vi "moveStageREL_xy.vi"(4 "Radio Buttons":enum32{"Coarse (mm) ", "Fine (um) "}(radio)=enum."Fine (um) ", 5 "increment":dbl, 6 "initPos (mm)":dbl, 7 "stage lim (mm)":dbl, 8 "axisIdx":i32, 9 "System no.":i32=1 min=1 max=4 step=1, 10 "stageInit":i16) -> (2 "finPos":dbl)   [LabVIEW 2015]
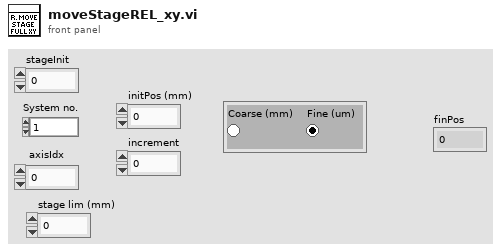
[diagram p1: front panel]
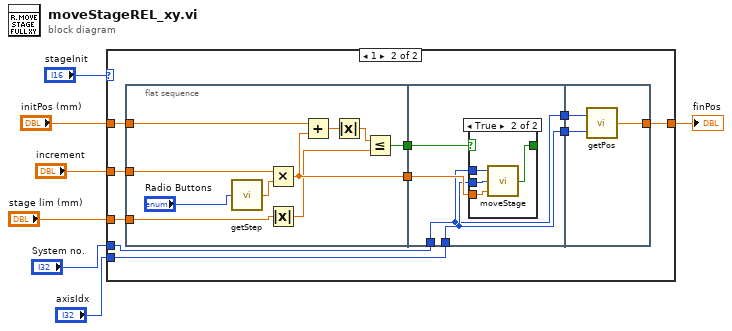
[diagram p0: block diagram]
diagram:
  n1 = case shown="1" "stageInit" {
    tunnel: [w8 w16] -> w7
    tunnel: "initPos (mm)" -> [w8 w13]
    tunnel: "System no." -> [_ w15]
    tunnel: "axisIdx" -> [_ w14]
    tunnel: "increment" -> [_ w12]
    tunnel: "stage lim (mm)" -> [_ w9]
    frame 0, Default {
    }
    frame 1 {
      n2 = flat-sequence {
        tunnel: [w27] -> w18
        tunnel: [w26] -> w17
        tunnel: w13 -> [w21]
        tunnel: w12 -> [w20]
        tunnel: w9 -> [w19]
        tunnel: w18 -> [w32]
        tunnel: w17 -> [w31]
        tunnel: w15 -> [w29]
        tunnel: w14 -> [w30]
        tunnel: [w30] -> w11
        tunnel: [w29] -> w10
        tunnel: [w40] -> w16
        tunnel: w11 -> [w39]
        tunnel: w10 -> [w38]
        frame #0 {
          n3 = call "getStep.vi"("Radio Buttons"="Radio Buttons") -> ("step"=w28:dbl)
          n4 = Multiply(x=w20, y=w28) -> (x*y=w26:dbl)
          n5 = Absolute Value(x=w19) -> (abs(x)=w23:dbl)
          n6 = Add(x=w21, y=w26) -> (x+y=w25:dbl)
          n7 = Absolute Value(x=w25) -> (abs(x)=w24:dbl)
          n8 = Less Or Equal?(x=w24, y=w23) -> (x <= y?=w27:bool)
        }
        frame #1 {
          n9 = case shown="True" w32 {
            selector: w32 -> [w33 _]
            tunnel: [w33 w37] -> _
            tunnel: w31 -> [_ w36]
            tunnel: w29 -> [_ w35]
            tunnel: w30 -> [_ w34]
            frame False {
            }
            frame True {
              n10 = call "moveStage.vi"("inc (mm)"=w36, "axisIdx"=w34, "System no."=w35) -> ("Stopped"=w37:bool)
            }
          }
        }
        frame #2 {
          n11 = call "getPos.vi"("axisIdx"=w39, "System no."=w38) -> ("stagePos"=w40:dbl)
        }
      }
    }
  }
  "finPos" <- w7
